vi "Post-Build Action.vi"(5 "Files Generated by Build":path[](array[path]), 6 "Top Level/Always Included VIs":path[](array[path]), 7 "Destination Path":path, 8 "error in (no error)":errorcluster, 9 "Target Name":string, 10 "Build Specification Name":string, 11 "Project Path":path) -> (0 "error out":errorcluster)   [LabVIEW 2020]
uses:
  <vilib>/AppBuilder/AB_API_Simple/Get Build Specification Version (path).vi
  <vilib>/AppBuilder/AB_API_Simple/NI_App_Builder_API.lvlib
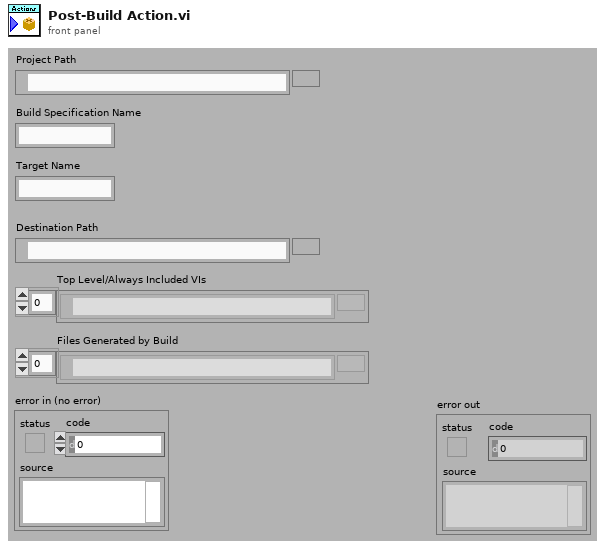
[diagram p1: front panel]
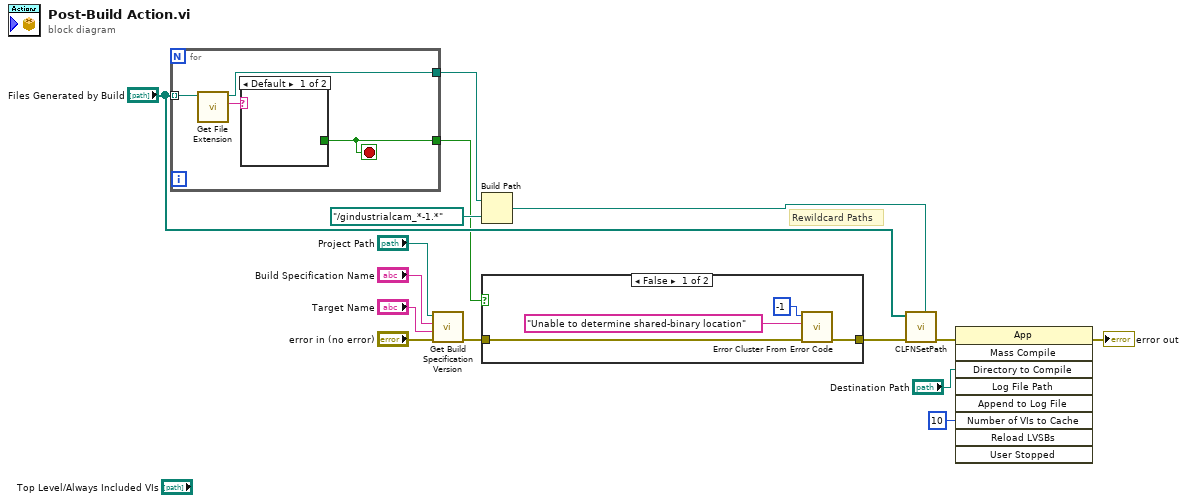
[diagram p0: block diagram]
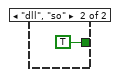
[diagram p3: hidden frame]
diagram:
  # "Rewildcard Paths"
  n1 = for {
    tunnel: "Files Generated by Build" -> [w19] mode=indexing
    tunnel: [w17] -> w9
    tunnel: [w16] -> w5
    stop <- w17 stop-if-true
    n2 = call <vilib>:"Get File Extension.vi"("file"=w19) -> ("lowercase file extension"=w18:string, "dup file"=w16:path)  [unwired: 6 in, 3 out]
    n3 = case shown="Default" w18 {
      tunnel: [_ TRUE] -> w17
      frame Default {
      }
      frame "dll", "so" {
      }
    }
  }
  n4 = call-poly <vilib>:"Get Build Specification Version.vi"("error in (no error)"="error in (no error)", "Name of target (My Computer)"="Target Name", "Name of build specification"="Build Specification Name", "Path to project"="Project Path") -> ("error out"=w8:errorcluster)  [unwired: 6 in, 1 out]
  n5 = Build Path(base path=w5, name or relative path=path "../gindustrialcam_*-1.*" ("New Path")) -> (appended path=w6:path)
  n6 = case shown="False" w9 {
    tunnel: w8 -> [w24 w25]
    tunnel: [w23 w25] -> w7
    frame False {
      n7 = call <vilib>:"Error Cluster From Error Code.vi"("error in (no error)"=w24, "error message (\"\")"="Unable to determine shared-binary location" ("error message (\"\")"), "error code (0)"=-1) -> ("error out"=w23:errorcluster)  [unwired: 6 in]
    }
    frame True {
    }
  }
  n8 = call "CLFNSetPath.vi"("New Path"=w6, "error in (no error)"=w7, "Files"="Files Generated by Build") -> ("error out"=w3:errorcluster)  [unwired: 7 in, 1 out]
  n9 = invoke class="App" method="Mass Compile"(error in=w3, "Directory to Compile"="Destination Path", "Number of VIs to Cache"=u32 10) -> (error out=→"error out":errorcluster)  [unwired: 6 in, 8 out]
